vi "Merge Image - Transform and Cast to U8.vi"(0 "Selected Image (U8 or U16)":T2[](array[typedef]), 1 "Dummy Image Ref":T2, 3 "Transform Parameters":T1[](array[typedef]) {"Image" items=["None"]}, 7 "RGB Image Refs (U8)":T2[](array[typedef]), 11 "RGB Image Refs (U16)":T2[](array[typedef])) -> (8 "RGB Image Refs (U8 DUP)":T2[](array[typedef]))   [LabVIEW 2016]
uses:
  <vilib>/vision/Image Controls.llb/IMAQ Image.ctl
  Merge Image Type Defs/Merge Image - Image Control.ctl
  <vilib>/vision/NI_Vision_Development_Module.lvlib
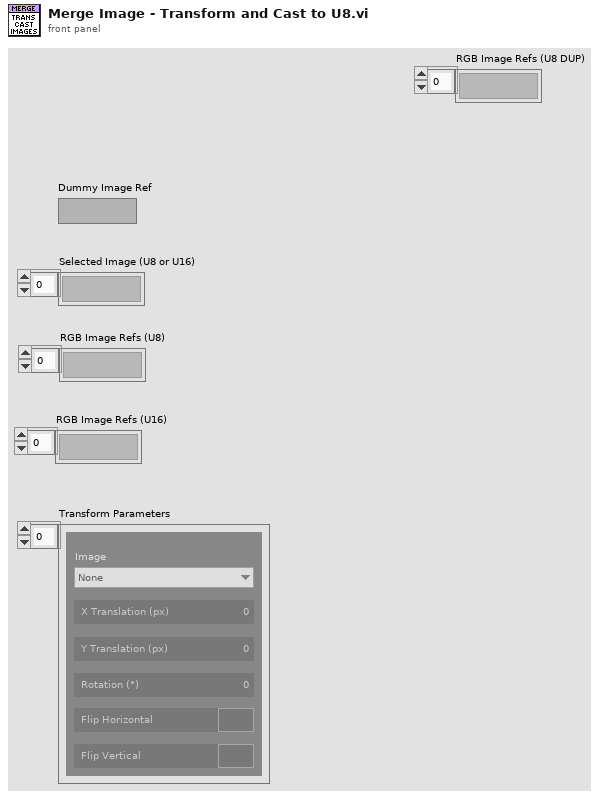
[diagram p1: front panel]
types:
  T1 = typedef "Merge Image - Image Control.ctl" = cluster{"Image":i32, "X Translation (px)":i32, "Y Translation (px)":i32, "Rotation (°)":sgl, "Flip Horizontal":bool, "Flip Vertical":bool}
  T2 = typedef "IMAQ Image.ctl" = refnum<image>
  T3 = typedef "Image Type" = u32
  T4 = cluster{"Mean Value":sgl, "Standard Variation":sgl, "Minimal Value":sgl, "Maximal Value":sgl, "Area (calibrated)":sgl, "Area (pixels)":u32, "%":sgl, "Calibration Valid":bool}
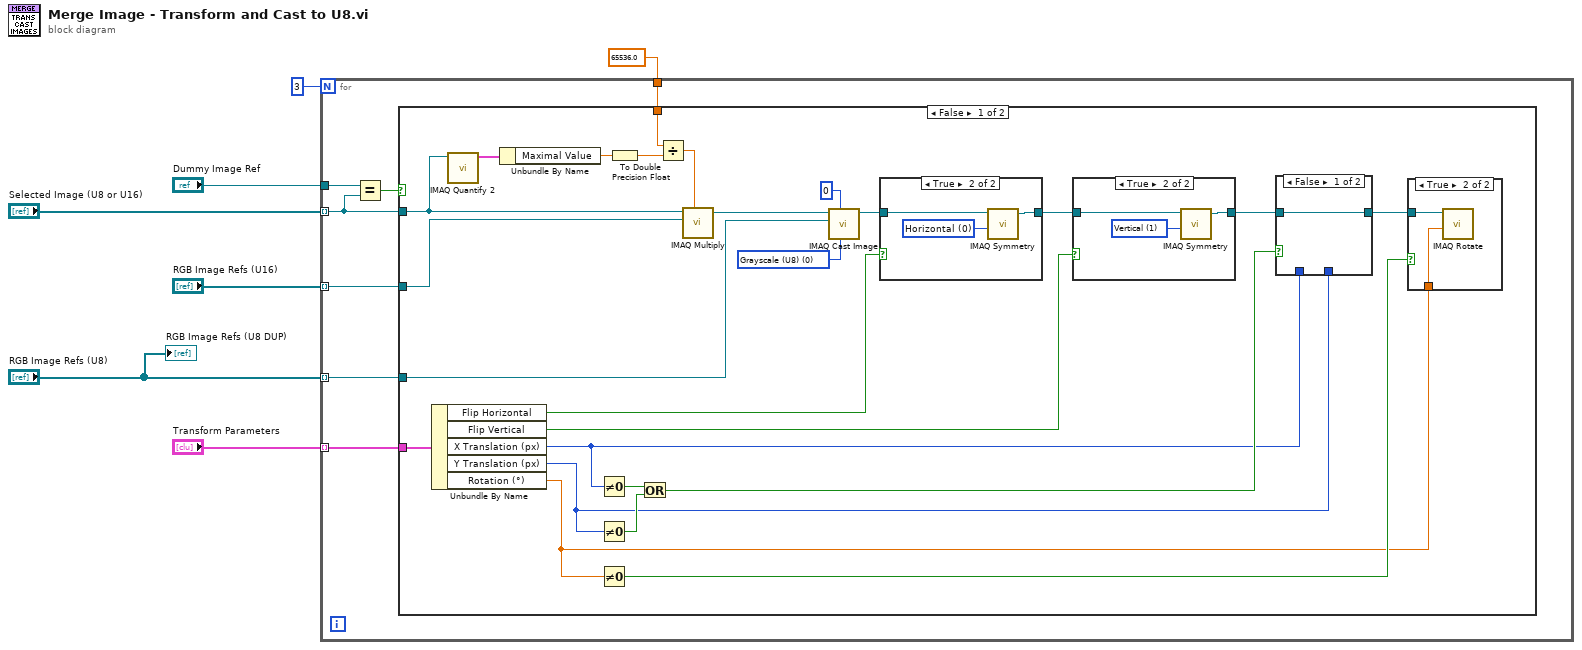
[diagram p0: block diagram]
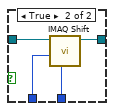
[diagram p3: hidden frame]
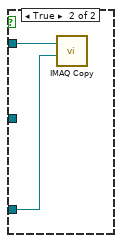
[diagram p6: hidden frame]
diagram:
  n1 = for {
    N: 3 -> [_]
    tunnel: "Selected Image (U8 or U16)" -> [w11] mode=indexing
    tunnel: "Dummy Image Ref" -> [w14]
    tunnel: "RGB Image Refs (U8)" -> [w12] mode=indexing
    tunnel: 65536.0 -> [w10]
    tunnel: "RGB Image Refs (U16)" -> [w9] mode=indexing
    tunnel: "Transform Parameters" -> [w8] mode=indexing
    n2 = Equal?(x=w14, y=w11) -> (x = y?=w13:bool)
    n3 = case shown="False" w13 {
      tunnel: w12 -> [w31 w55]
      tunnel: w11 -> [w35 w56]
      tunnel: w10 -> [w36 _]
      tunnel: w9 -> [w33 _]
      tunnel: w8 -> [w28 _]
      frame False {
        w29 = T3 0 items=["Grayscale (U8)", "Grayscale (I16)", "Grayscale (SGL)", "Complex (CSG)", "RGB (U32)", "HSL (U32)", "RGB (U64)", "Grayscale (U16)"] ("Image Type")
        n4 = Unbundle By Name(w28) -> ("Flip Horizontal"=w26:bool, "Flip Vertical"=w24:bool, "X Translation (px)"=w19:i32, "Y Translation (px)"=w18:i32, "Rotation (°)"=w15:sgl)
        n5 = call "IMAQ Quantify 2"("Image"=w35) -> ("Global Report"=w37:T4)  [unwired: 8 in, 2 out]
        n6 = Unbundle By Name(w37) -> ("Maximal Value"=w38:sgl)
        n7 = Not Equal To 0?(x=w19) -> (x != 0?=w23:bool)
        n8 = Not Equal To 0?(x=w18) -> (x != 0?=w22:bool)
        n9 = Not Equal To 0?(x=w15) -> (x != 0?=w17:bool)
        n10 = To Double Precision Float(number=w38) -> (double precision float=w39:dbl)
        n11 = Or(x=w23, y=w22) -> (x .or. y?=w21:bool)
        n12 = Divide(x=w36, y=w39) -> (x/y=w34:dbl)
        n13 = call "IMAQ Multiply"("Image Src A"=w35, "Constant"=w34, "Image Dst"=w33) -> ("Image Dst Out"=w32:T2)  [unwired: 4 in, 1 out]
        n14 = call "IMAQ Cast Image"("Image Type"=w29, "# Shifts"=0, "Image Dst"=w31, "Image Src"=w32) -> ("Image Dst Out"=w27:T2)  [unwired: 6 in, 1 out]
        n15 = case shown="True" w26 {
          tunnel: w27 -> [w51 w54]
          tunnel: [w51 w52] -> w25
          frame False {
          }
          frame True {
            w53 = u32 0 items=["Horizontal", "Vertical", "Central", "1st Diagonal", "2nd Diagonal"] ("Type of Symmetry")
            n16 = call "IMAQ Symmetry"("Type of Symmetry"=w53, "Image Src"=w54) -> ("Image Dst Out"=w52:T2)  [unwired: 3 in, 1 out]
          }
        }
        n17 = case shown="True" w24 {
          tunnel: w25 -> [w47 w50]
          tunnel: [w47 w48] -> w20
          frame False {
          }
          frame True {
            w49 = u32 1 items=["Horizontal", "Vertical", "Central", "1st Diagonal", "2nd Diagonal"] ("Type of Symmetry")
            n18 = call "IMAQ Symmetry"("Type of Symmetry"=w49, "Image Src"=w50) -> ("Image Dst Out"=w48:T2)  [unwired: 3 in, 1 out]
          }
        }
        n19 = case shown="False" w21 {
          tunnel: w20 -> [w42 w46]
          tunnel: w19 -> [_ w45]
          tunnel: w18 -> [_ w44]
          tunnel: [w42 w43] -> w16
          frame False {
          }
          frame True {
            n20 = call "IMAQ Shift"("YOffset"=w44, "XOffset"=w45, "Image Src"=w46) -> ("Image Dst Out"=w43:T2)  [unwired: 7 in, 1 out]
          }
        }
        n21 = case shown="True" w17 {
          tunnel: w16 -> [_ w41]
          tunnel: w15 -> [_ w40]
          frame False {
          }
          frame True {
            n22 = call "IMAQ Rotate"("Angle (degrees)"=w40, "Image Src"=w41) -> ()  [unwired: 8 in, 2 out]
          }
        }
      }
      frame True {
        n23 = call "IMAQ Copy"("Image Dst"=w55, "Image Src"=w56) -> ()  [unwired: 4 in, 2 out]
      }
    }
  }
  "RGB Image Refs (U8 DUP)" <- "RGB Image Refs (U8)"
